vi "Save Excel(mass).vi"(0 "Master Report Path":path, 1 "Protected?":bool, 2 "Password":string, 3 "Filter":bool, 7 "Save Path":path, 12 "eData":T1(array[cluster]), 13 "OK":bool, 14 "Close?":bool) -> (8 "Saved?":bool, 15 "error out":errorcluster)   [LabVIEW 2020]
uses:
  <vilib>/Utility/miscctls.llb/LVPointTypeDef.ctl
  <vilib>/addons/_office/NI_ReportGenerationToolkit.lvlib
  <vilib>/Utility/NIReport.llb/Excel/NI_Excel.lvclass
panel:
  out "Report Saved %":dbl(slide) scale=0.0..100.0 scale format="%#_6f"
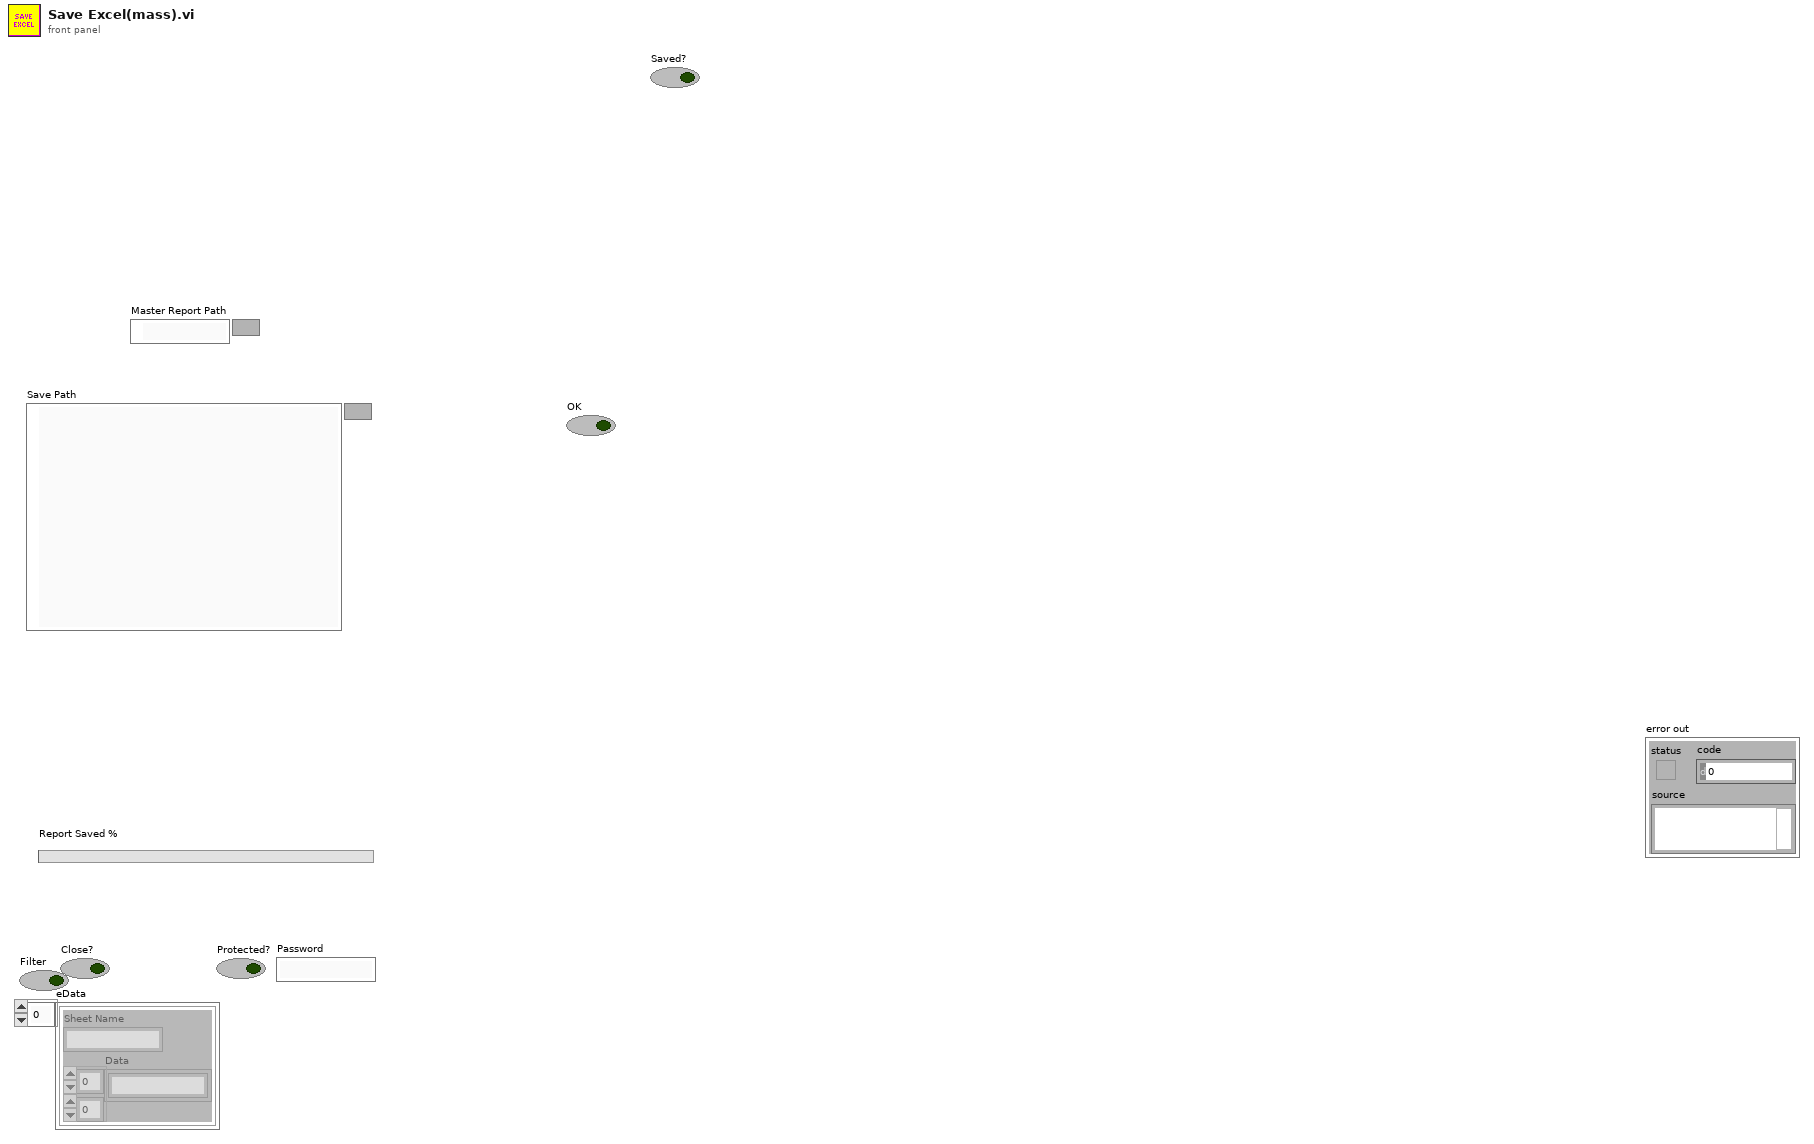
[diagram p1: front panel]
types:
  T1 = cluster{"Sheet Name":string, "Data":string[][]}[]
  T2 = typedef "LVPointTypeDef.ctl" = cluster{"Horizontal":i16, "Vertical":i16}
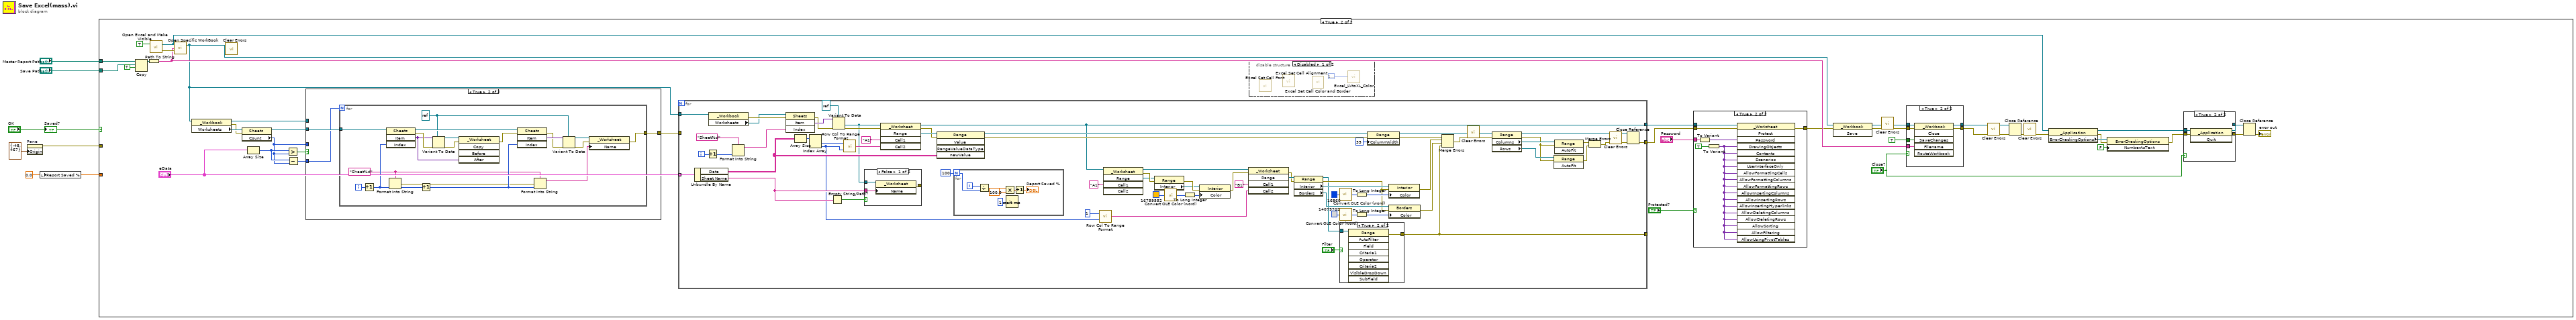
[diagram p0: block diagram]
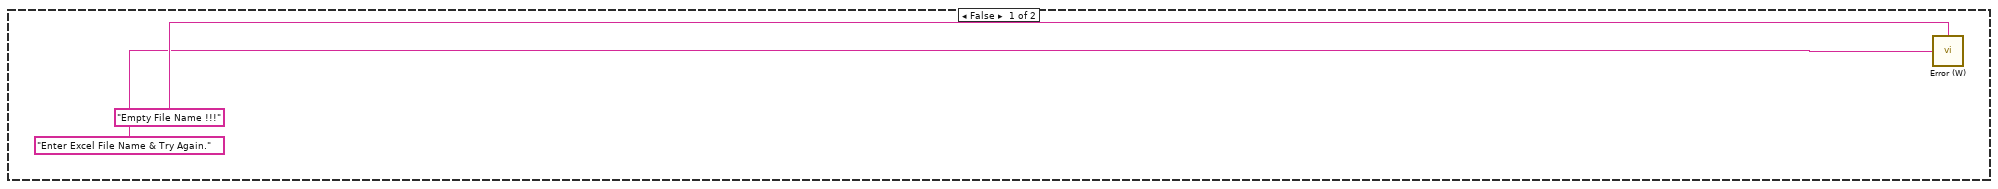
[diagram p2: hidden frame]
diagram:
  w3 = 0.0 ("Report Saved %")
  n1 = property on="Pane" class="Pane"("Origin"=T2 {"Horizontal"=-48, "Vertical"=467} ("Origin 2")) -> (error out=w1:errorcluster)  [unwired: 2 in, 1 out]
  n2 = local write "Report Saved %"(w3) -> ()
  n3 = case shown="True" "OK" {
    tunnel: "Save Path" -> [_ w48]
    tunnel: "Master Report Path" -> [_ w47]
    tunnel: w3 -> [_ _]
    tunnel: w1 -> [_ _]
    frame False {
      n4 = call <userlib>:"Error (W).vi"("Title"="Empty File Name !!!" ("Control Name"), "Warning in"="Enter Excel File Name & Try Again." ("Control Name")) -> ()  [unwired: 14 in]
    }
    frame True {
      n5 = Copy(9:TRUE ("overwrite (F)"), 10:w48, 11:w47) -> (3:w45:path)  [unwired: 2 in, 2 out]
      n6 = Path To String(path=w45) -> (string=w35:string)
      n7 = call <userlib>:"Open Excel and Make Visible.vi"("Visible Boolean"=TRUE) -> ("error out"=w49:errorcluster, "Excel._Application"=w23:refnum<k7>)  [unwired: 1 in]
      n8 = call <userlib>:"Open Specific WorkBook.vi"("error in (no error)"=w49, "Filename of Workbook"=w35, "Excel._Application"=w23) -> ("Excel._Workbook"=w21:refnum<k7>)  [unwired: 1 out]
      n9 = property class="_Workbook"(reference=w21) -> (reference out=w11:refnum<k7>, error out=w19:errorcluster, "Worksheets"=w20:refnum<k7>)  [unwired: 1 in]
      n10 = call <vilib>:"Clear Errors.vi"() -> ()  [unwired: 6 in, 2 out]
      n11 = property class="Sheets"(reference=w20, error in=w19) -> (reference out=w16:refnum<k7>, "Count"=w14:i32)  [unwired: 1 out]
      n12 = Array Size(array="eData") -> (size(s)=w15:i32)
      n13 = Greater?(x=w15, y=w14) -> (0:w17:bool)
      n14 = Subtract(x=w15, y=w14) -> (x-y=w13:i32)
      n15 = case shown="True" w17 {
        tunnel: w16 -> [_ w53]
        tunnel: w14 -> [_ _]
        tunnel: w13 -> [_ w52]
        tunnel: [_ w54] -> w12
        tunnel: w11 -> [_ _]
        frame False {
        }
        frame True {
          n16 = for {
            N: w52 -> [_]
            tunnel: [w66] -> w54
            tunnel: w53 -> [w73]
            i -> [w72]
            w56 = refnum<k7> refnum ("Excel._Worksheet")
            w55 = "Sheet%d" ("Sheet")
            n17 = Increment(x=w72) -> (x+1=w62:i32)
            n18 = invoke class="Sheets" method="Item"(reference=w73, "Index"=w62) -> (reference out=w57:refnum<k7>, error out=w63:errorcluster, "Item"=w59:variant)  [unwired: 2 in, 1 out]
            n19 = Format Into String(format string=w55, w62) -> (error out=w65:errorcluster)  [unwired: 2 in, 1 out]
            n20 = Increment(x=w62) -> (x+1=w68:i32)
            n21 = Variant To Data(error in=w63, type=w56, Variant=w59) -> (data=w60:refnum<k7>, error out=w58:errorcluster)
            n22 = invoke class="_Worksheet" method="Copy"(reference=w60, error in=w58, "After"=w59) -> (error out=w71:errorcluster)  [unwired: 2 in, 4 out]
            n23 = invoke class="Sheets" method="Item"(reference=w57, error in=w71, "Index"=w68) -> (error out=w69:errorcluster, "Item"=w70:variant)  [unwired: 1 in, 2 out]
            n24 = Format Into String(format string=w55, error in=w65, w68) -> (resulting string=w67:string)  [unwired: 1 in, 1 out]
            n25 = Variant To Data(error in=w69, type=w56, Variant=w70) -> (data=w61:refnum<k7>, error out=w64:errorcluster)
            n26 = property class="_Worksheet"(reference=w61, error in=w64, "Name"=w67) -> (error out=w66:errorcluster)  [unwired: 1 out]
          }
        }
      }
      n27 = for {
        tunnel: w21 -> [w135]
        tunnel: [w74] -> w30
        tunnel: [w132] -> w29
        tunnel: "eData" -> [w126] mode=indexing
        tunnel: w12 -> [_]
        tunnel: [w86] -> _
        i -> [w123]
        n28 = Unbundle By Name(w126) -> ("Data"=w125:string[][], "Sheet Name"=w118:string)
        n29 = Increment(x=w123) -> (x+1=w122:i32)
        n30 = property class="_Workbook"(reference=w135) -> (error out=w134:errorcluster, "Worksheets"=w133:refnum<k7>)  [unwired: 1 in, 1 out]
        n31 = Format Into String(format string="Sheet%d" ("Sheet"), w122) -> (resulting string=w121:string)  [unwired: 2 in, 1 out]
        n32 = invoke class="Sheets" method="Item"(reference=w133, error in=w134, "Index"=w121) -> (error out=w141:errorcluster, "Item"=w142:variant)  [unwired: 1 in, 2 out]
        n33 = Array Size(array=w125) -> (size(s)=w137:i32[])
        n34 = Index Array(array=w137) -> (element #1=w129:i32, element #2=w101:i32)  [unwired: 2 in]
        n35 = Empty String/Path?(string/path=w118) -> (empty?=w119:bool)
        n36 = Variant To Data(error in=w141, type=refnum<k7> refnum ("Excel._Worksheet"), Variant=w142) -> (data=w120:refnum<k7>, error out=w140:errorcluster)
        n37 = call <userlib>:"Row Col To Range Format.vi"("Column"=w101, "Row"=w129) -> ("Output String"=w130:string)
        n38 = case shown="False" w119 {
          tunnel: w120 -> [w148 _]
          tunnel: w118 -> [w147 _]
          tunnel: [w146 _] -> _
          frame False {
            n39 = property class="_Worksheet"(reference=w148, "Name"=w147) -> (error out=w146:errorcluster)  [unwired: 1 in, 1 out]
          }
          frame True {
          }
        }
        n40 = invoke class="_Worksheet" method="Range"(reference=w120, error in=w140, "Cell1"="A1" ("Cell"), "Cell2"=w130) -> (reference out=w74:refnum<k7>, error out=w138:errorcluster, "Range"=w139:refnum<k7>)  [unwired: 1 in, 2 out]
        n41 = invoke class="Range" method="Value"(reference=w139, error in=w138, "newValue"=w125) -> (reference out=w83:refnum<k7>, error out=w81:errorcluster)  [unwired: 2 in, 3 out]
        n42 = for {
          N: 100 -> [w152]
          i -> [w151]
          n43 = Divide(x=w151, y=w152) -> (x/y=w154:dbl)
          n44 = Multiply(x=w154, y=100.0) -> (x*y=w155:dbl)
          n45 = Wait (ms)(milliseconds to wait=u32 1) -> ()  [unwired: 1 out]
          n46 = Increment(x=w155) -> (x+1=→"Report Saved %":dbl)
        }
        n47 = call <userlib>:"Row Col To Range Format.vi"("Column"=w101, "Row"=1) -> ("Output String"=w99:string)
        n48 = invoke class="_Worksheet" method="Range"(reference=w74, "Cell1"="A1" ("Cell")) -> (reference out=w103:refnum<k7>, error out=w116:errorcluster, "Range"=w114:refnum<k7>)  [unwired: 3 in, 2 out]
        n49 = property class="Range"(reference=w114, error in=w116) -> (error out=w115:errorcluster, "Interior"=w113:refnum<k7>)  [unwired: 1 out]
        n50 = call <vilib>:"Convert OLE Color (word).vi"("color in"=u32 16759552 ("Selection Color")) -> ("color out"=w112:u32)
        n51 = To Long Integer(number=w112) -> (32bit integer=w110:i32)
        n52 = property class="Interior"(reference=w113, error in=w115, "Color"=w110) -> (error out=w102:errorcluster)  [unwired: 1 out]
        n53 = invoke class="_Worksheet" method="Range"(reference=w103, error in=w102, "Cell1"="B1" ("Cell"), "Cell2"=w99) -> (error out=w98:errorcluster, "Range"=w105:refnum<k7>)  [unwired: 1 in, 3 out]
        n54 = property class="Range"(reference=w105, error in=w98) -> (reference out=w91:refnum<k7>, error out=w93:errorcluster, "Interior"=w106:refnum<k7>, "Borders"=w97:refnum<k7>)
        n55 = call <vilib>:"Convert OLE Color (word).vi"("color in"=u32 16860 ("Selection Color")) -> ("color out"=w107:u32)
        n56 = call <vilib>:"Convert OLE Color (word).vi"("color in"=u32 14079702 ("Selection Color")) -> ("color out"=w96:u32)
        n57 = case shown="True" "Filter" {
          tunnel: w91 -> [_ w145]
          tunnel: [_ w144] -> w86
          frame False {
          }
          frame True {
            n58 = invoke class="Range" method="AutoFilter"(reference=w145) -> (error out=w144:errorcluster)  [unwired: 8 in, 8 out]
          }
        }
        n59 = To Long Integer(number=w107) -> (32bit integer=w109:i32)
        n60 = To Long Integer(number=w96) -> (32bit integer=w94:i32)
        n61 = property class="Range"(reference=w83, error in=w81, "ColumnWidth"=35 ("Row")) -> (reference out=w82:refnum<k7>, error out=w80:errorcluster)
        n62 = property class="Interior"(reference=w106, error in=w93, "Color"=w109) -> (error out=w88:errorcluster)  [unwired: 1 out]
        n63 = property class="Borders"(reference=w97, error in=w93, "Color"=w94) -> (error out=w87:errorcluster)  [unwired: 1 out]
        n64 = Merge Errors(w80, w88, w87, w86) -> (w89:errorcluster)
        n65 = call <vilib>:"Clear Errors.vi"("error in (no error)"=w89) -> ("error out"=w85:errorcluster)  [unwired: 5 in, 1 out]
        n66 = property class="Range"(reference=w82, error in=w85) -> (reference out=w92:refnum<k7>, error out=w77:errorcluster, "Columns"=w84:refnum<k7>, "Rows"=w78:refnum<k7>)
        n67 = invoke class="Range" method="AutoFit"(reference=w78, error in=w77) -> (error out=w75:errorcluster)  [unwired: 1 in, 2 out]
        n68 = invoke class="Range" method="AutoFit"(reference=w84, error in=w77) -> (error out=w128:errorcluster)  [unwired: 1 in, 2 out]
        n69 = Merge Errors(w128, w75) -> (w76:errorcluster)
        n70 = call <vilib>:"Clear Errors.vi"("error in (no error)"=w76) -> ("error out"=w127:errorcluster)  [unwired: 5 in, 1 out]
        n71 = Close Reference(reference=w92, error in (no error)=w127) -> (error out=w132:errorcluster)
      }
      n72 = disable-structure shown="Disabled" {
        frame Disabled {
          n73 = call <vilib>:"Excel Set Cell Font.vi"() -> ()  [unwired: 14 in, 2 out]
          n74 = call <vilib>:"Excel Set Cell Alignment.vi"() -> ()  [unwired: 14 in, 2 out]
          n75 = call <vilib>:"Excel Set Cell Color and Border.vi"() -> ()  [unwired: 14 in, 2 out]
          n76 = call <vilib>:"Excel_LVtoXL_Color.vi"("LabVIEW color"=u32 16777226 ("Selection Color")) -> ()  [unwired: 1 out]
        }
        frame Enabled {
        }
      }
      n77 = case shown="True" "Protected?" {
        tunnel: w30 -> [_ w163]
        tunnel: w29 -> [w156 w162]
        tunnel: [w156 w161] -> w34
        tunnel: "Password" -> [_ w160]
        frame False {
        }
        frame True {
          n78 = To Variant(anything=w160) -> (Variant=w159:variant)
          n79 = To Variant(anything=TRUE ("Close?")) -> (Variant=w157:variant)
          n80 = invoke class="_Worksheet" method="Protect"(reference=w163, error in=w162, "Password"=w159, "DrawingObjects"=w157, "Contents"=w157, "Scenarios"=w157, "UserInterfaceOnly"=w157, "AllowFormattingCells"=w157, "AllowFormattingColumns"=w157, "AllowFormattingRows"=w157, "AllowInsertingColumns"=w157, "AllowInsertingRows"=w157, "AllowInsertingHyperlinks"=w157, "AllowDeletingColumns"=w157, "AllowDeletingRows"=w157, "AllowSorting"=w157, "AllowFiltering"=w157, "AllowUsingPivotTables"=w157) -> (error out=w161:errorcluster)  [unwired: 1 in, 18 out]
        }
      }
      n81 = invoke class="_Workbook" method="Save"(reference=w21, error in=w34) -> (reference out=w40:refnum<k7>, error out=w9:errorcluster)  [unwired: 1 in, 1 out]
      n82 = call <vilib>:"Clear Errors.vi"("error in (no error)"=w9) -> ("error out"=w39:errorcluster)  [unwired: 5 in, 1 out]
      n83 = case shown="True" "Close?" {
        tunnel: w40 -> [w165 w171]
        tunnel: [w164 w169] -> w38
        tunnel: [w165 w170] -> w31
        tunnel: w39 -> [w164 w168]
        tunnel: TRUE ("Close?") -> [_ w167]
        tunnel: w35 -> [_ w166]
        frame False {
        }
        frame True {
          n84 = invoke class="_Workbook" method="Close"(reference=w171, error in=w168, "SaveChanges"=w167, "Filename"=w166) -> (reference out=w170:refnum<k7>, error out=w169:errorcluster)  [unwired: 2 in, 4 out]
        }
      }
      n85 = call <vilib>:"Clear Errors.vi"("error in (no error)"=w38) -> ("error out"=w10:errorcluster)  [unwired: 5 in, 1 out]
      n86 = Close Reference(reference=w31, error in (no error)=w10) -> (error out=w43:errorcluster)
      n87 = call <vilib>:"Clear Errors.vi"("error in (no error)"=w43) -> ("error out"=w26:errorcluster)  [unwired: 5 in, 1 out]
      n88 = property class="_Application"(reference=w23, error in=w26) -> (reference out=w22:refnum<k7>, error out=w27:errorcluster, "ErrorCheckingOptions"=w28:refnum<k7>)
      n89 = property class="ErrorCheckingOptions"(reference=w28, error in=w27, "NumberAsText"=FALSE) -> (error out=w25:errorcluster)  [unwired: 1 out]
      n90 = case shown="True" "Close?" {
        tunnel: w22 -> [w173 w177]
        tunnel: w25 -> [w172 w176]
        tunnel: [w172 w175] -> w42
        tunnel: [w173 w174] -> w41
        frame False {
        }
        frame True {
          n91 = invoke class="_Application" method="Quit"(reference=w177, error in=w176) -> (reference out=w174:refnum<k7>, error out=w175:errorcluster)  [unwired: 1 in, 1 out]
        }
      }
      n92 = Close Reference(reference=w41, error in (no error)=w42) -> (error out=→"error out":errorcluster)
    }
  }
  "Saved?" <- "OK"
